vi "Read Continuous B Sweep.json.vi"(8 "error in (no error)":errorcluster, 10 "file (use dialog)":path, 11 "SweepControl in":refnum<class "Sweep Control.lvclass">) -> (0 "error out":errorcluster, 3 "SweepControl out":refnum<class "Sweep Control.lvclass">)   [LabVIEW 2019, in "Sweep Control.lvclass"]
uses:
  Sweep Control.lvclass
  <userlib>/LevyLab/Transport/Control Experiment/Typedefs/Wiring Description--cluster.ctl
  <userlib>/LevyLab/Transport/Control Experiment/Control Experiment.lvclass
  <userlib>/LevyLab/Transport/Control Experiment/Typedefs/Experiment Description--cluster.ctl
  Typedefs/Enum - Experiments.ctl
  Typedefs/Continuous B Sweep JSON--Cluster.ctl
  <userlib>/LevyLab/Lockin-Multichannel/Instrument.DAQ/Typedefs/REF.Channel--Cluster--Array.ctl
  <userlib>/LevyLab/Lockin-Multichannel/Instrument.DAQ/Instrument.DAQ.lvclass
  <userlib>/LevyLab/Lockin-Multichannel/Instrument.DAQ/Typedefs/AO.Channel--Cluster--Array.ctl
  4a7b423a-b6d0-49b2-a88e-35961dfeee01.vi
  <userlib>/LevyLab/Transport/Control Experiment/Typedefs/Instruments--cluster.ctl
  <userlib>/LevyLab/Krohn Hite 7008/KH7008/typedefs/Filter--Enum.ctl
  <userlib>/LevyLab/Krohn Hite 7008/KH7008/KH7008.lvlib
  <userlib>/LevyLab/Krohn Hite 7008/KH7008/typedefs/couple--Enum.ctl
  <userlib>/LevyLab/Krohn Hite 7008/KH7008/typedefs/shunt--enum.ctl
  <userlib>/LevyLab/Krohn Hite 7008/KH7008/typedefs/Input--Enum.ctl
  <userlib>/LevyLab/Krohn Hite 7008/KH7008/typedefs/gain--enum.ctl
  <userlib>/LevyLab/Krohn Hite 7008/KH7008/typedefs/channel--numeric.ctl
  <userlib>/LevyLab/Krohn Hite 7008/KH7008/typedefs/channelProperties--Cluster.ctl
  <userlib>/LevyLab/Krohn Hite 7008/KH7008/typedefs/allChannelProperties--Array.ctl
  <userlib>/LevyLab/Lockin-Multichannel/Instrument.DAQ/Typedefs/AO.Channel.Function--Enum.ctl
  <userlib>/LevyLab/Lockin-Multichannel/Instrument.DAQ/Typedefs/AO.Channel--Cluster.ctl
  <userlib>/LevyLab/Lockin-Multichannel/Instrument.DAQ/Typedefs/REF.Channel--Cluster.ctl
  <userlib>/LevyLab/Transport/Control Experiment/Typedefs/Instrument Types--enum.ctl
panel:
  out "ContinuousBSweep":T1={"Continuous B Sweep"={"Experiment"=enum."Lockin_DelayLine", "B field values"=[]}, "Experiment Description"={"User"="", "Device"="", "Device Path"=path "", "Device Description"="", "Experiment Path"=path "", "Experiment Description"="", "Instrument"="", "Instruments"=[], "Sweep"=[]}, "Wiring Configuration"={"Lockin Ch"=[], "KH"={"Electrodes"=[], "Labels"=[]}, "not KH"={"Electrodes"=[], "Labels"=[]}}, "Lockin"={"AOconfig"=[], "REFconfig"=[]}, "Krohn Hite"={"Channel Setting"=[]}} {"Krohn Hite"."Channel Setting"."channel" min=1 max=8 step=1; "Lockin"."REFconfig"."Roll-Off" min=1; "Lockin"."REFconfig"."TC" min=0.0001 format="%#_3p"; "Lockin"."REFconfig"."Phase" format="%.3g"; "Lockin"."REFconfig"."Frequency" min=0.0001 max=10000.0 format="%.3g"; "Lockin"."REFconfig"."Channel" min=1; "Lockin"."AOconfig"."Phase" format="%.2g"; "Lockin"."AOconfig"."Frequency" min=0.0001 max=10000.0 format="%.2g"; "Lockin"."AOconfig"."Offset" format="%5.2p"; "Lockin"."AOconfig"."Amplitude" min=0.0 max=10.0 format="%5.2p"}
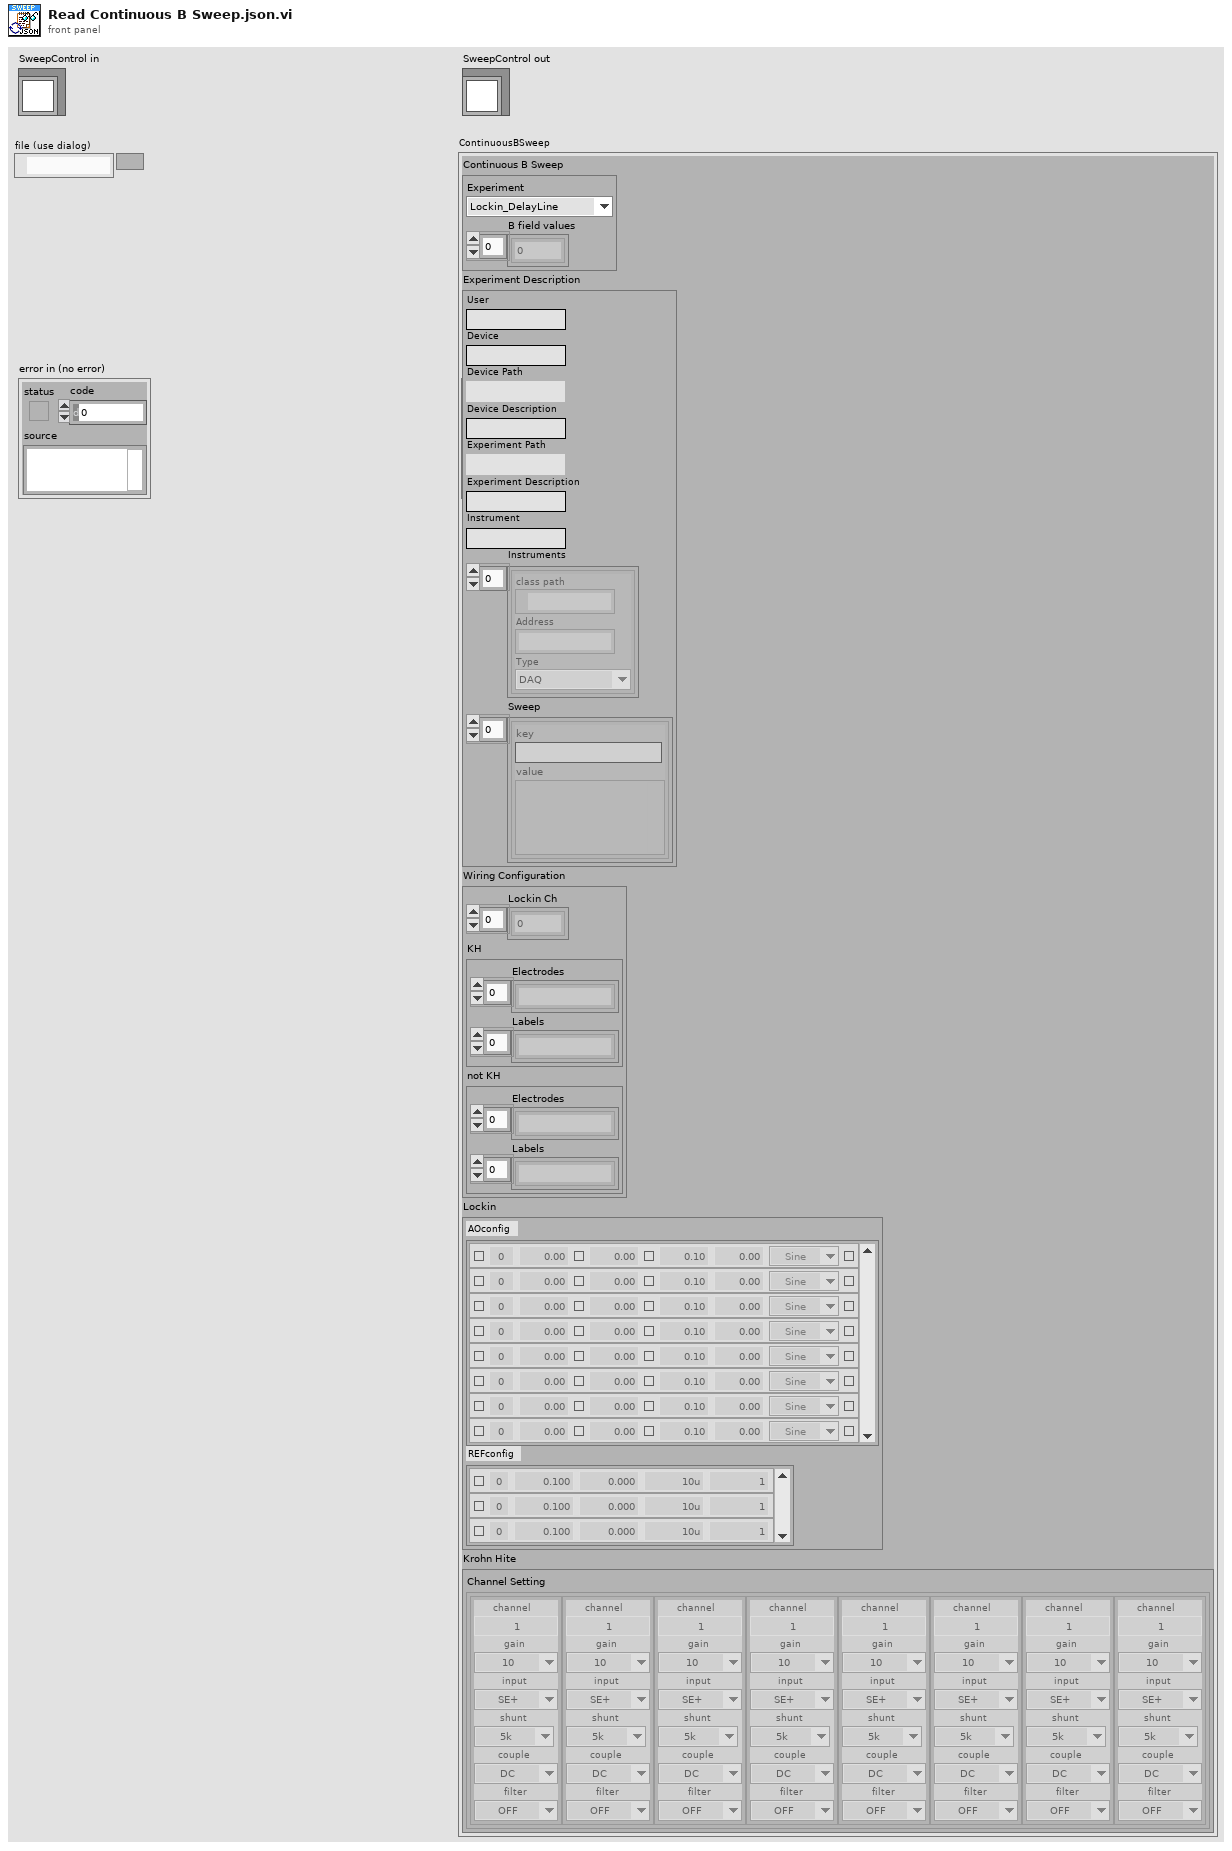
[diagram p1: front panel]
types:
  T1 = typedef "Sweep Control.lvclass/Continuous B Sweep JSON--Cluster.ctl" = cluster{"Continuous B Sweep":cluster{"Experiment":T2, "B field values":dbl[]}, "Experiment Description":T3, "Wiring Configuration":T6, "Lockin":cluster{"AOconfig":T7, "REFconfig":T10}, "Krohn Hite":cluster{"Channel Setting":T12}}
  T2 = typedef "Sweep Control.lvclass/Enum - Experiments.ctl" = enum16{"Lockin_time", "Lockin_sweep", "Lockin_DelayLine"}
  T3 = typedef "Control Experiment.lvclass/Experiment Description--cluster.ctl" = cluster{"User":string, "Device":string, "Device Path":path, "Device Description":string, "Experiment Path":path, "Experiment Description":string, "Instrument":string, "Instruments":T4[], "Sweep":cluster{"key":string, "value":variant}[]}
  T4 = typedef "Control Experiment.lvclass/Instruments--cluster.ctl" = cluster{"class path":path, "Address":string, "Type":T5}
  T5 = typedef "Control Experiment.lvclass/Instrument Types--enum.ctl" = enum16{"DAQ", "Amplifier", "Temperature", "Magnet", "Rotator", "Level", "Capacitance", "Delay Line", "Strain Cell", "VNA", "Source"}
  T6 = typedef "Control Experiment.lvclass/Wiring Description--cluster.ctl" = cluster{"Lockin Ch":i32[], "KH":cluster{"Electrodes":string[], "Labels":string[]}, "not KH":cluster{"Electrodes":string[], "Labels":string[]}}
  T7 = typedef "Instrument.Lockin.lvlib/Instrument.DAQ.lvclass/AO.Channel--Cluster--Array.ctl" = T8[]
  T8 = typedef "Instrument.Lockin.lvlib/Instrument.DAQ.lvclass/AO.Channel--Cluster.ctl" = cluster{"Enable?":bool, "Channel":i32, "Amplitude":dbl, "Offset":dbl, "Frequency":dbl, "Phase":dbl, "Function":T9, "Sweeping?":bool, "Limit AC":bool, "Limit DC?":bool}
  T9 = typedef "Instrument.Lockin.lvlib/Instrument.DAQ.lvclass/AO.Channel.Function--Enum.ctl" = enum16{"Sine", "Triangle", "Square"}
  T10 = typedef "Instrument.Lockin.lvlib/Instrument.DAQ.lvclass/REF.Channel--Cluster--Array.ctl" = T11[]
  T11 = typedef "Instrument.Lockin.lvlib/Instrument.DAQ.lvclass/REF.Channel--Cluster.ctl" = cluster{"Enable?":bool, "Channel":i32, "Frequency":dbl, "Phase":dbl, "TC":dbl, "Roll-Off":i32}
  T12 = typedef "KH7008.lvlib/allChannelProperties--Array.ctl" = T13[]
  T13 = typedef "KH7008.lvlib/channelProperties--Cluster.ctl" = cluster{"channel":T14, "gain":T15, "input":T16, "shunt":T17, "couple":T18, "filter":T19}
  T14 = typedef "KH7008.lvlib/channel--numeric.ctl" = u16
  T15 = typedef "KH7008.lvlib/gain--enum.ctl" = enum16{"1", "10", "100", "1000"}
  T16 = typedef "KH7008.lvlib/input--enum.ctl" = enum16{"OFF", "SE+", "SE-", "DIFF"}
  T17 = typedef "KH7008.lvlib/shunt--enum.ctl" = enum16{"Open", "50", "500", "5k", "50k", "10M"}
  T18 = typedef "KH7008.lvlib/couple--enum.ctl" = enum16{"AC", "DC"}
  T19 = typedef "KH7008.lvlib/filter--enum.ctl" = enum16{"OFF", "ON"}
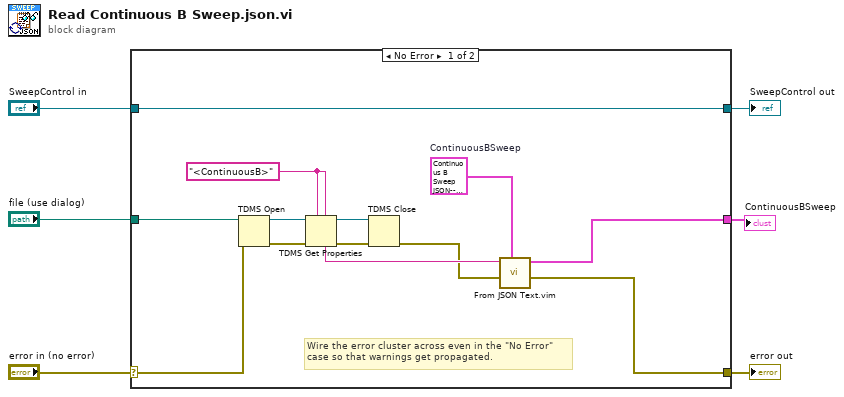
[diagram p0: block diagram]
diagram:
  n1 = case shown="No Error" "error in (no error)" {
    selector: "error in (no error)" -> [w13 w21]
    tunnel: [w7 w21] -> w5
    tunnel: [w19 w20] -> w3
    tunnel: "SweepControl in" -> [w19 w20]
    tunnel: "file (use dialog)" -> [w14 _]
    tunnel: [w8 _] -> w1
    frame No Error {
      w18 = "<ContinuousB>" ("group name")
      w9 = T1 {"Continuous B Sweep"={"Experiment"=enum."Lockin_DelayLine", "B field values"=[]}, "Experiment Description"={"User"="", "Device"="", "Device Path"=path "", "Device Description"="", "Experiment Path"=path "", "Experiment Description"="", "Instrument"="", "Instruments"=[], "Sweep"=[]}, "Wiring Configuration"={"Lockin Ch"=[], "KH"={"Electrodes"=[], "Labels"=[]}, "not KH"={"Electrodes"=[], "Labels"=[]}}, "Lockin"={"AOconfig"=[], "REFconfig"=[]}, "Krohn Hite"={"Channel Setting"=[]}}  # ContinuousBSweep
      # "Wire the error cluster across even in the \"No Error\"\ncase so that warnings get propagated."
      n2 = TDMS Open(8:w13, 11:w14) -> (0:w12:errorcluster, 3:w17:refnum<k34>)  [unwired: 5 in]
      n3 = TDMS Get Properties(5:w18, 7:w18, 8:w12, 11:w17) -> (0:w11:errorcluster, 3:w16:refnum<k34>, 4:w15:string)  [unwired: 2 in, 3 out]
      n4 = TDMS Close(8:w11, 11:w16) -> (0:w10:errorcluster)  [unwired: 1 out]
      n5 = call "From JSON Text.vim"("Data Type and Default Value"=w9, "error in (no error)"=w10, "JSON"=w15) -> ("error out"=w7:errorcluster, "Data out"=w8:T1)  [unwired: 7 in]
    }
    frame Error {
    }
  }
  "error out" <- w5
  "SweepControl out" <- w3
  "ContinuousBSweep" <- w1
